vi "GetTraceName.vi"(8 "error in (no error)":errorcluster, 11 "SpecAnBase in":refnum<class "SpecAnBase.lvclass">) -> (0 "error out":errorcluster, 2 "TraceName":string[](array[string]), 3 "SpecAnBase out":refnum<class "SpecAnBase.lvclass">)   [LabVIEW 2018, in "SpecAnPlugins.lvlib" / "SpecAnBase.lvclass"]
doc: "This function returns the specific driver defined trace name that corresponds to the index that the user specifies. If the driver defines a qualified trace name, this property returns the qualified name. If the value that the user passes for the Index parameter is less than one or greater than the value of the Trace Count attribute, the function returns an empty string in the Name parameter and returns the Invalid Value error."
uses:
  SpecAnBase.lvclass
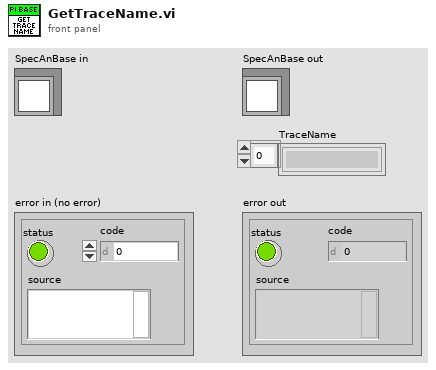
[diagram p1: front panel]
types:
  T1 = typedef "SpecAnPlugins.lvlib/SpecAnBase.lvclass/Trace.ctl" = cluster{"TraceName":string, "TraceSize":i32, "TraceType":enum16{"Clear Write", "Maximum Hold", "Minimum Hold", "Video Average", "View", "Store"}}[]
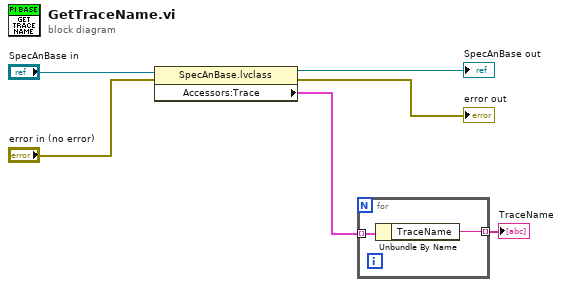
[diagram p0: block diagram]
diagram:
  n1 = property class="SpecAnBase.lvclass"(reference="SpecAnBase in", error in="error in (no error)") -> (reference out=→"SpecAnBase out":refnum<class "SpecAnBase.lvclass">, error out=→"error out":errorcluster, "Accessors:Trace"=w2:T1)
  n2 = for {
    tunnel: w2 -> [w8] mode=indexing
    tunnel: [w7] -> w1 mode=indexing
    n3 = Unbundle By Name(w8) -> ("TraceName"=w7:string)
  }
  "TraceName" <- w1
